vi "PenaltyAttackTacticVSS.vi"(6 "States":enum16{"PenaltyPos", "Exit"}(ring), 9 "Game in":refnum<class "Game.lvclass">, 10 "Robot":refnum<class "Robot.lvclass">, 11 "PenaltyAttackTacticVSS in":refnum<class "PenaltyAttackTacticVSS.lvclass">) -> (2 "Robot out":refnum<class "Robot.lvclass">, 3 "PenaltyAttackTacticVSS out":refnum<class "PenaltyAttackTacticVSS.lvclass">)   [LabVIEW 2018, in "PenaltyAttackTacticVSS.lvclass"]
uses:
  PenaltyAttackTacticVSS.lvclass
  C:/Users/anton/Desktop/RoboIme/vsspssl/SSL_AI/Tactic_class/Tactic.lvclass
  Robot_class/Robot.lvclass
  Game_class/Game.lvclass
  Tactic_class/Tactic.lvclass/Tactic.ctl
  Robot_class/tactics.ctl
  Robot_class/Robot.lvclass/Robot.ctl
  Tactic_class/Read Skillbook.vi
  Robot_class/Write tactic.vi
  Skillbook_class/Skillbook.lvclass
  KickSkillVSS_class/KickSkillVSS.lvclass
  PenaltyPosSkillVSS_class/PenaltyPosSkillVSS.lvclass
  BallDispPosSkillVSS_class/BallDispPosSkillVSS.lvclass
  BallToGoalSkillVSS_class/BallToGoalSkillVSS.lvclass
  GoToBallSkillVSS_class/GoToBallSkillVSS.lvclass
  DefBallPosSkillVSS_class/DefBallPosSkillVSS.lvclass
  HaltSkill_class/HaltSkill.lvclass
panel:
  out "x .or. y?":bool
  out "error out 2":errorcluster
  in  "error in (no error) 2":errorcluster
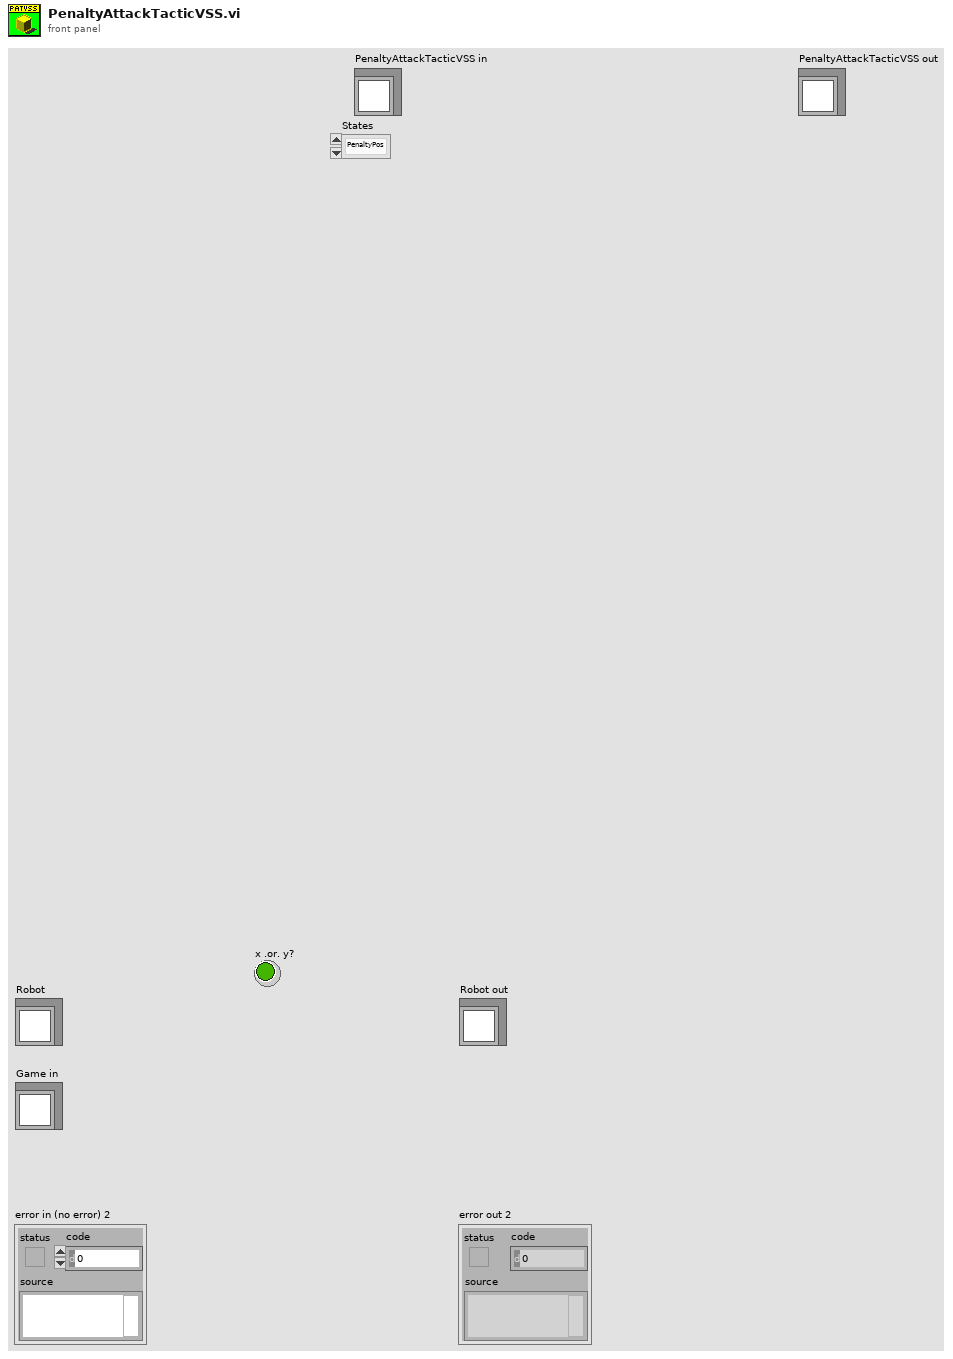
[diagram p1: front panel]
types:
  T1 = typedef "tactics.ctl" = enum16{"ReceivePassInFuturePoint", "Roller", "PrepareRollToPassRollerGoTo", "PrepareRollToPassReceiverGoTo", "WaitRoll", "PositionToRoll", "PenaltyAttacker", "PassObserver", "PenaltyDefense", "TableReceiverTactic", "Test", "DefendGoal", "Marker", "FollowAttacker", "DefendArea", "Shoot", "AttackerAimGoal", "AttackerBallOutOfField", "AttackerBlock", "AttackerStop", "Duelist", "Halt", "ZigZag", "GoTo", "Timeout", "KickToPassReceiver", "PositionToReceivePass", "DefendAreaVSS", "DefendGoalVSS", "KickVSS", "AttackVSS", "DispBallVSS", "PenaltyAttackVSS", "WaitPass"}
  T2 = cluster{"KickSkillVSS":refnum<class "KickSkillVSS.lvclass">, "PenaltyPosSkillVSS":refnum<class "PenaltyPosSkillVSS.lvclass">, "BallDispPosSkillVSS":refnum<class "BallDispPosSkillVSS.lvclass">, "BallToGoalSkillVSS":refnum<class "BallToGoalSkillVSS.lvclass">, "GoToBallSkillVSS":refnum<class "GoToBallSkillVSS.lvclass">, "DefBallPosSkillVSS":refnum<class "DefBallPosSkillVSS.lvclass">, "HaltSkill":refnum<class "HaltSkill.lvclass">}
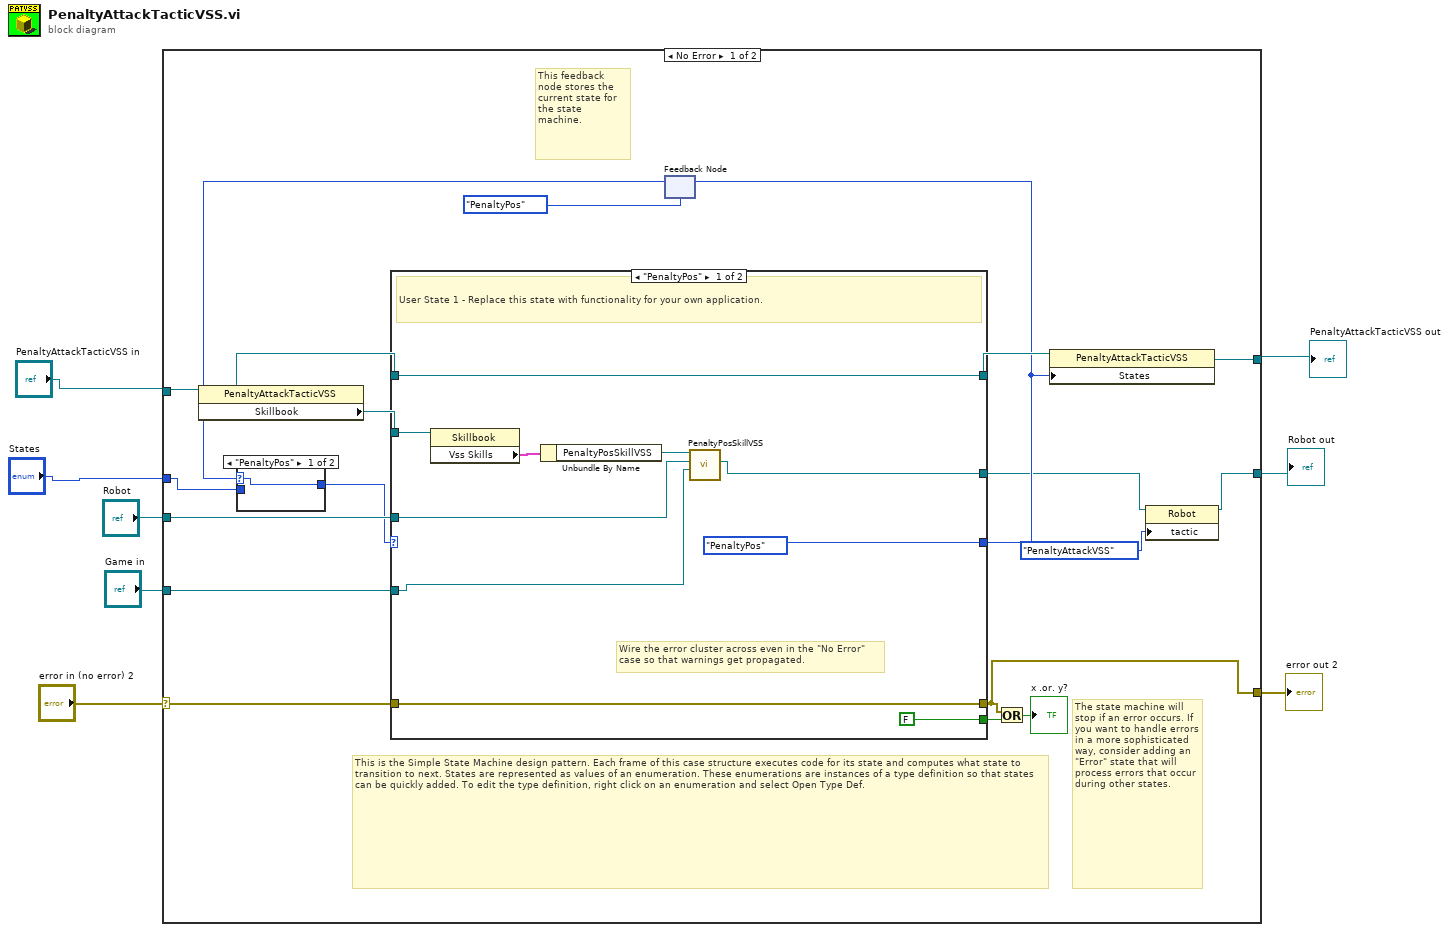
[diagram p0: block diagram]
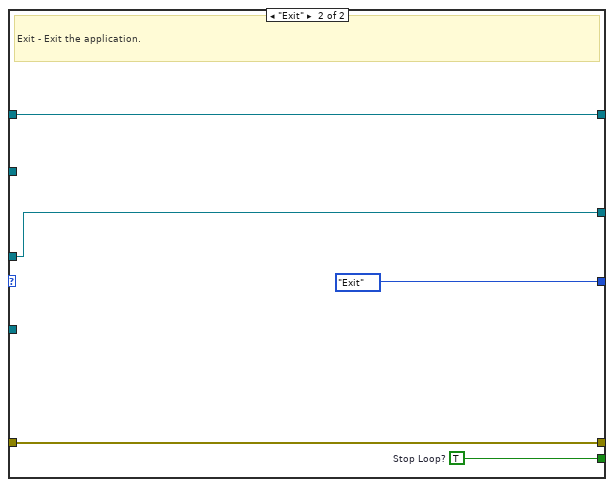
[diagram p3: hidden frame]
diagram:
  n1 = case shown="No Error" "error in (no error) 2" {
    selector: "error in (no error) 2" -> [w19 w46]
    tunnel: [w18 w46] -> w7
    tunnel: [w16 w45] -> w2
    tunnel: "PenaltyAttackTacticVSS in" -> [w22 w45]
    tunnel: "Robot" -> [w21 w44]
    tunnel: "Game in" -> [w20 _]
    tunnel: [w10 w44] -> w4
    tunnel: "States" -> [w13 _]
    frame No Error {
      # "The state machine will stop if an error occurs. If you want to handle errors in a more sophisticated way, consider adding an \"Error\" state that will process errors that occur during other states."
      # "This feedback node stores the current state for the state machine."
      # "This is the Simple State Machine design pattern. Each frame of this case structure executes code for its state and computes what state to transition to next. States are represented as values of an enumeration. These enumerations are instances of a type definition so that states can be quickly added. To edit the type definition, right click on an enumeration and select Open Type Def."
      # "Wire the error cluster across even in the \"No Error\"\ncase so that warnings get propagated."
      n2 = property class="PenaltyAttackTacticVSS"(reference=w22) -> ("Skillbook"=w24:refnum<class "Skillbook.lvclass">)  [unwired: 1 in, 2 out]
      n3 = feedback #1(enum16{"PenaltyPos", "Exit"}."PenaltyPos" ("States")) -> (w15:enum16{"PenaltyPos", "Exit"})
      n4 = case shown="\"PenaltyPos\"" w15 {
        selector: w15 -> [w27 _]
        tunnel: [w27 w28] -> w14
        tunnel: w13 -> [_ w28]
        frame "PenaltyPos" {
        }
        frame "Exit" {
        }
      }
      n5 = case shown="\"PenaltyPos\"" w14 {
        tunnel: [enum16{"PenaltyPos", "Exit"}."PenaltyPos" ("States") enum16{"PenaltyPos", "Exit"}."Exit" ("States")] -> w17
        tunnel: [FALSE ("Stop Loop?") w43] -> w26
        tunnel: w24 -> [w37 _]
        tunnel: w21 -> [w31 w42]
        tunnel: [w29 w42] -> w11
        tunnel: [w36 w41] -> w23
        tunnel: w22 -> [w36 w41]
        tunnel: w20 -> [w30 _]
        tunnel: [w35 w40] -> w18
        tunnel: w19 -> [w35 w40]
        frame "PenaltyPos" {
          # "User State 1 - Replace this state with functionality for your own application."
          n6 = property class="Skillbook"(reference=w37) -> ("Vss Skills"=w33:T2)  [unwired: 1 in, 2 out]
          n7 = Unbundle By Name(w33) -> ("PenaltyPosSkillVSS"=w32:refnum<class "PenaltyPosSkillVSS.lvclass">)
          n8 = call-dynamic "PenaltyPosSkillVSS.vi"("Game"=w30, "Robot in"=w31, "PenaltyPosSkillVSS in"=w32) -> ("Robot out"=w29:refnum<class "Robot.lvclass">)  [unwired: 6 in, 2 out]
        }
        frame "Exit" {
          w43 = TRUE  # Stop Loop?
          # "Exit - Exit the application."
        }
      }
      n9 = feedback-in #1(w17) -> ()
      n10 = Or(x=w18, y=w26) -> (x .or. y?=→"x .or. y?":bool)
      n11 = property class="PenaltyAttackTacticVSS"(reference=w23, "States"=w17) -> (reference out=w16:refnum<class "PenaltyAttackTacticVSS.lvclass">)  [unwired: 1 in, 1 out]
      n12 = property class="Robot"(reference=w11, "tactic"=tactics."PenaltyAttackVSS") -> (reference out=w10:refnum<class "Robot.lvclass">)  [unwired: 1 in, 1 out]
    }
    frame Error {
    }
  }
  "PenaltyAttackTacticVSS out" <- w2
  "error out 2" <- w7
  "Robot out" <- w4
